vi "SupportedHardware.vi"() -> (1 "Channels per Module":i32[](array[numeric])=[3, 3, 3, 4, 4], 3 "Supported Hardware":string[](array[string]))   [LabVIEW 2017, in "CmsAcquisition.lvlib"]
uses:
  <vilib>/addons/InsightCM/Devices/Shared/Cms/CmsAcquisition/CmsAcquisition.lvlib
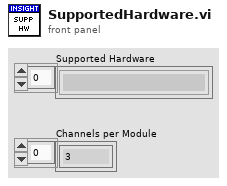
[diagram p1: front panel]
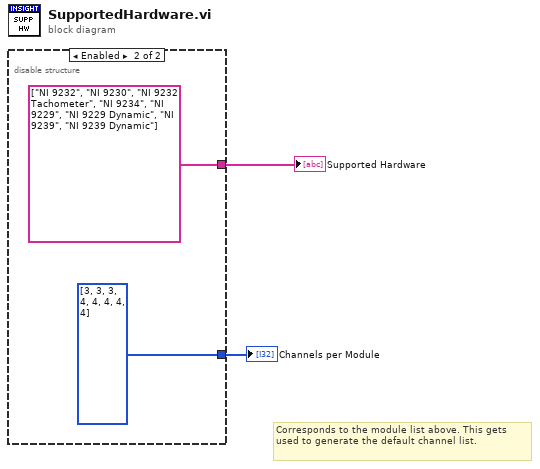
[diagram p0: block diagram]
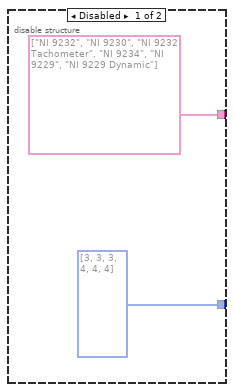
[diagram p2: hidden frame]
diagram:
  # "Corresponds to the module list above. This gets used to generate the default channel list."
  n1 = disable-structure shown="Enabled" {
    disable-tunnel: [string[] ["NI 9232", "NI 9230", "NI 9232 Tachometer", "NI 9234", "NI 9229", "NI 9229 Dynamic"] string[] ["NI 9232", "NI 9230", "NI 9232 Tachometer", "NI 9234", "NI 9229", "NI 9229 Dynamic", "NI 9239", "NI 9239 Dynamic"]] -> w2
    disable-tunnel: [i32[] [3, 3, 3, 4, 4, 4] i32[] [3, 3, 3, 4, 4, 4, 4, 4]] -> w1
    frame Disabled {
    }
    frame Enabled {
    }
  }
  "Supported Hardware" <- w2
  "Channels per Module" <- w1
